vi "Initialize_DBL.vi"(8 "error in (no error)":errorcluster, 10 "Angle (degrees)":dbl, 11 "PolarVector in":refnum<class "PolarVector.lvclass">) -> (0 "error out":errorcluster, 3 "PolarVector out":refnum<class "PolarVector.lvclass">)   [LabVIEW 2011, in "PolarVector.lvclass"]
uses:
  PolarVector.lvclass
  Angles/Angle/Angle.lvclass
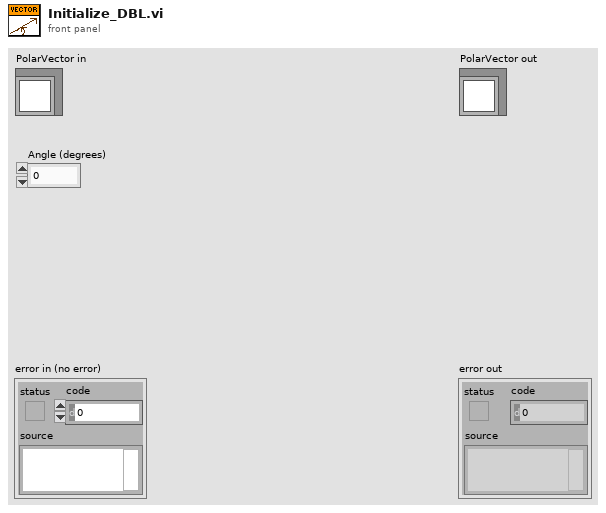
[diagram p1: front panel]
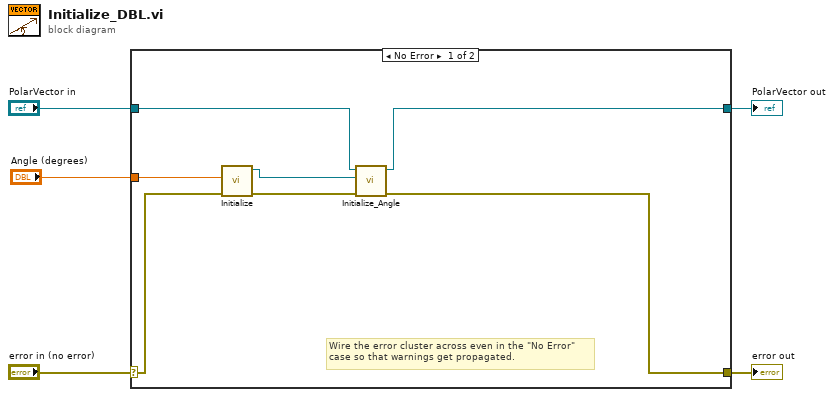
[diagram p0: block diagram]
diagram:
  n1 = case shown="No Error" "error in (no error)" {
    selector: "error in (no error)" -> [w12 w14]
    tunnel: [w10 w14] -> w4
    tunnel: [w6 w13] -> w2
    tunnel: "PolarVector in" -> [w7 w13]
    tunnel: "Angle (degrees)" -> [w9 _]
    frame No Error {
      # "Wire the error cluster across even in the \"No Error\"\ncase so that warnings get propagated."
      n2 = call "Initialize.vi"("error in (no error)"=w12, "Input Angle (Deg.)"=w9) -> ("error out"=w11:errorcluster, "Angle out"=w8:refnum<class "Angle.lvclass">)  [unwired: 8 in]
      n3 = call "Initialize_Angle.vi"("error in (no error)"=w11, "Angle.lvclass"=w8, "PolarVector in"=w7) -> ("error out"=w10:errorcluster, "PolarVector out"=w6:refnum<class "PolarVector.lvclass">)  [unwired: 7 in]
    }
    frame Error {
    }
  }
  "error out" <- w4
  "PolarVector out" <- w2
